vi "local variables-while loop.vi"() -> ()   [LabVIEW 2013]
panel:
  out "Boolean 2":bool
  in  "stop":bool
  out "Boolean":bool
  in  "LED switch":bool
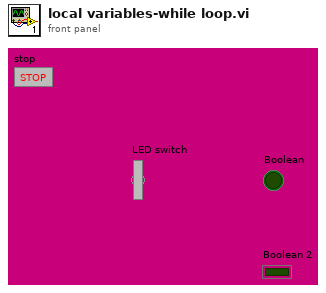
[diagram p1: front panel]
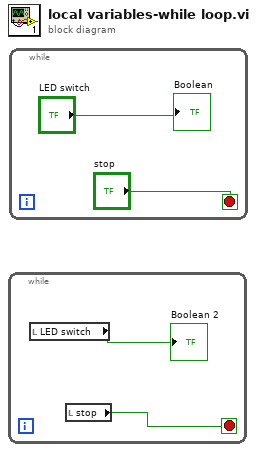
[diagram p0: block diagram]
diagram:
  n1 = while {
    stop <- w2 stop-if-true
    n2 = local read "LED switch"() -> (→"Boolean 2":bool)
    n3 = local read "stop"() -> (w2:bool)
  }
  n4 = while {
    stop <- "stop" stop-if-true
    "Boolean" <- "LED switch"
  }
